vi "Test_WriteMixedTypes_ReadWithFilter_ReturnMatchedType.vi"(8 "error in (no error)":errorcluster, 11 "TestCase in":refnum<class "TestComposedLookupTable.lvclass">) -> (0 "error out":errorcluster, 3 "TestCase out":refnum<class "TestComposedLookupTable.lvclass">)   [LabVIEW 2017, in "TestComposedLookupTable.lvclass"]
uses:
  TestComposedLookupTable.lvclass
  Source/LookupTable/LookupTable.lvclass/LookupTable.ctl
  a70eb062-d5c1-4dd5-a9a5-4b40db1fd60a.vi
  4b67c015-f057-4287-88ec-8a8209823235.vi
  7e646295-b973-4596-a171-731298737383.vi
  aebfe81e-859d-4b55-8554-9e41685d696a.vi
  Source/LookupTable/Read Table Reference.vi
  a70eb062-d5c1-4dd5-a9a5-4b40db1fd60a.vi/8bda7c28-8b06-4bb2-90d0-9514a2f79d85.vi
  4b67c015-f057-4287-88ec-8a8209823235.vi/cbe8392d-8948-4258-8b8d-2d22d31cf8f9.vi
  7e646295-b973-4596-a171-731298737383.vi/1d6ef6d4-ab8b-4edb-86df-b01ea4cdb99f.vi
  Source/LookupTable/LookupTable.lvclass
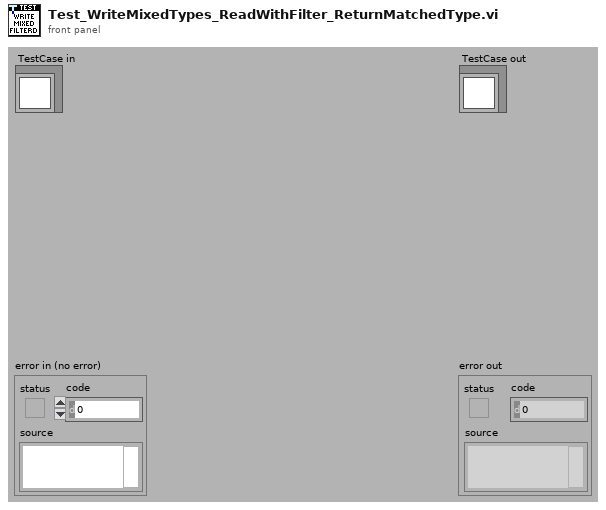
[diagram p1: front panel]
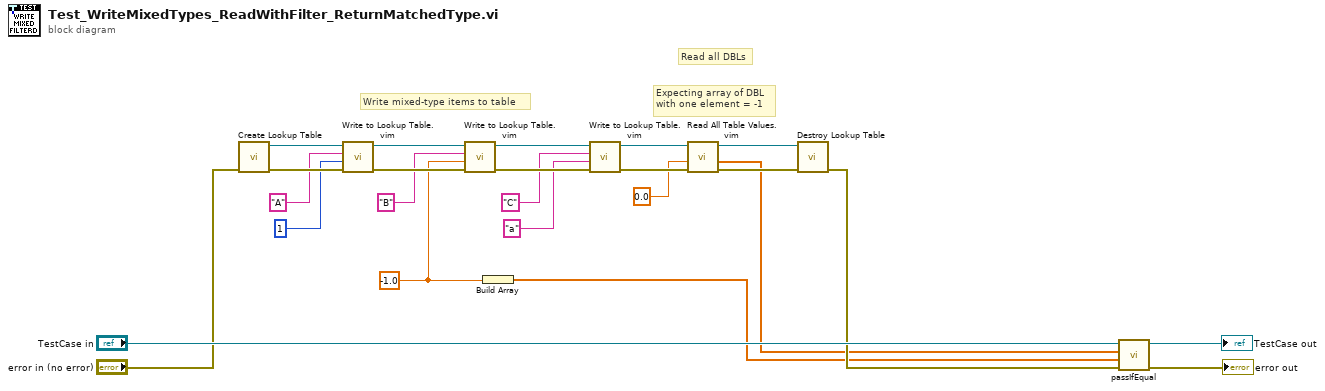
[diagram p0: block diagram]
diagram:
  w2 = -1.0
  # "Read all DBLs"
  # "Expecting array of DBL\nwith one element = -1"
  # "Write mixed-type items to table"
  n1 = call "Create Lookup Table.vi"("error in (no error)"="error in (no error)") -> ("error out"=w23:errorcluster, "LookupTable Reference"=w16:refnum<data-value>)  [unwired: 9 in]
  n2 = call "Write to Lookup Table.vim"("error in (no error)"=w23, "Item"=1, "Item Name"="A", "LookupTable Reference"=w16) -> ("error out"=w18:errorcluster, "LookupTable Reference Out"=w19:refnum<data-value>)  [unwired: 5 in, 1 out]
  n3 = call "Write to Lookup Table.vim"("error in (no error)"=w18, "Item"=w2, "Item Name"="B", "LookupTable Reference"=w19) -> ("error out"=w24:errorcluster, "LookupTable Reference Out"=w11:refnum<data-value>)  [unwired: 5 in, 1 out]
  n4 = Build Array(w2) -> (w1:dbl[])
  n5 = call "Write to Lookup Table.vim"("error in (no error)"=w24, "Item"="a", "Item Name"="C", "LookupTable Reference"=w11) -> ("error out"=w10:errorcluster, "LookupTable Reference Out"=w8:refnum<data-value>)  [unwired: 5 in, 1 out]
  n6 = call "Read All Table Values.vim"("error in (no error)"=w10, "Type (All)"=0.0, "LookupTable Reference"=w8) -> ("error out"=w9:errorcluster, "Values"=w6:dbl[], "LookupTable Reference Out"=w7:refnum<data-value>)  [unwired: 5 in, 1 out]
  n7 = call "Destroy Lookup Table.vi"("error in (no error)"=w9, "LookupTable Reference"=w7) -> ("error out"=w14:errorcluster)  [unwired: 9 in]
  n8 = call-dynamic "passIfEqual.vi"("error in (no error)"=w14, "y"=w1, "x"=w6, "TestCase in"="TestCase in") -> ("error out"=→"error out":errorcluster, "TestCase out"=→"TestCase out":refnum<class "TestComposedLookupTable.lvclass">)  [unwired: 6 in]
